vi "Temperature Simulator.vi"(11 "entrée d'erreur (pas d'erreur)":errorcluster) -> (6 "Graphe":dynamicdata(graph) caption="Waveform Graph", 15 "sortie d'erreur":errorcluster)   [LabVIEW 2009]
doc: "Ce VI simule une génération de température sous forme de génération de tension continue + bruit avec un échantillonnage de 50 kHz et 5000 points. Ce VI sert de simulation dans le projet Station météo si aucun matériel n'est disponible."
uses:
  Instance           1 29Saved   Temperature Simulator .vi
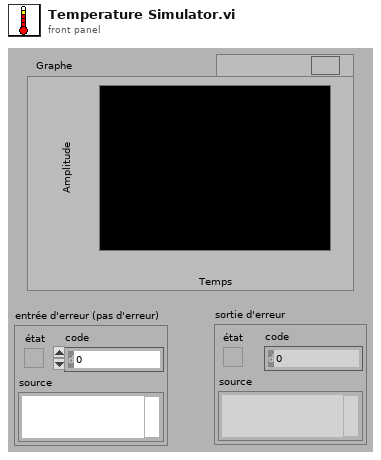
[diagram p1: front panel]
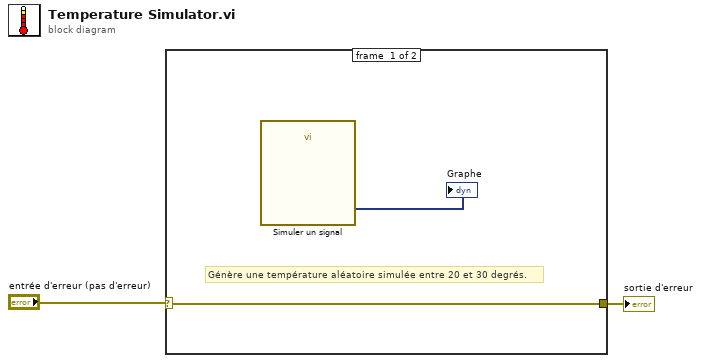
[diagram p0: block diagram]
diagram:
  n1 = case "Structure Condition" shown="Pas d'erreur" "entrée d'erreur (pas d'erreur)" {
    selector: "entrée d'erreur (pas d'erreur)" -> [w4 w5]
    tunnel: [w4 w5] -> w1
    frame #0 {
      # "Génère une température aléatoire simulée entre 20 et 30 degrés."
      n2 = call "Simuler un signal"() -> ("Température"=→"Graphe":dynamicdata)  [unwired: 5 in, 10 out]
    }
    frame #1 {
    }
  }
  "sortie d'erreur" <- w1
